vi "Mech Drive.vi"(11 "JoystickDevRef":T1) -> (3 "motor values":dbl[](array[numeric]))   [LabVIEW 2018]
uses:
  <vilib>/Rock Robotics/WPI/Joystick/WPI_JoystickDevRef.ctl
  <vilib>/Rock Robotics/WPI/Joystick/WPI_JoystickDeviceEnum.ctl
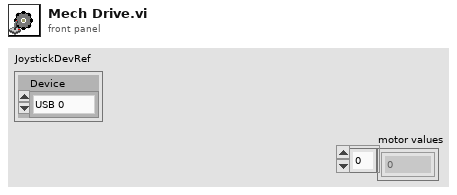
[diagram p1: front panel]
types:
  T1 = typedef "WPI_JoystickDevRef.ctl" = cluster{"Device":T2}
  T2 = typedef "WPI_JoystickDeviceEnum.ctl" = enum16{"USB 0", "USB 1", "USB 2", "USB 3", "USB 4", "USB 5"}
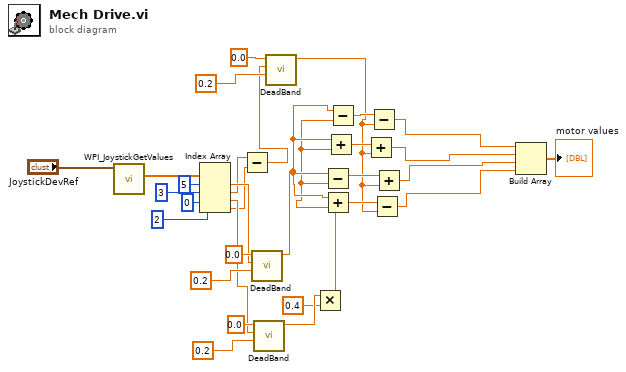
[diagram p0: block diagram]
diagram:
  n1 = call <vilib>:"WPI_JoystickGetValues.vi"("JoystickDevRef"="JoystickDevRef") -> ("Axes"=w30:dbl[])  [unwired: 6 in, 4 out]
  n2 = Index Array(array=w30, index #1=5 ("index"), index #2=3 ("index"), index #3=0 ("index"), index #4=2 ("index")) -> (element #1=w11:dbl, element #2=w7:dbl, element #3=w10:dbl, element #4=w6:dbl)
  n3 = Subtract(x=w7, y=w6) -> (x-y=w5:dbl)
  n4 = call "DeadBand.vi"("Threshold"=0.2, "Process Variable"=w11, "Send Value"=0.0) -> ("Output"=w4:dbl)  [unwired: 7 in, 1 out]
  n5 = call "DeadBand.vi"("Threshold"=0.2, "Process Variable"=w10, "Send Value"=0.0) -> ("Output"=w2:dbl)  [unwired: 7 in, 1 out]
  n6 = call "DeadBand.vi"("Threshold"=0.2, "Process Variable"=w5, "Send Value"=0.0) -> ("Output"=w17:dbl)  [unwired: 7 in, 1 out]
  n7 = Multiply(x=w2, y=0.4) -> (x*y=w3:dbl)
  n8 = Subtract(x=w4, y=w3) -> (x-y=w25:dbl)
  n9 = Add(x=w4, y=w3) -> (x+y=w24:dbl)
  n10 = Add(x=w4, y=w3) -> (x+y=w26:dbl)
  n11 = Subtract(x=w4, y=w3) -> (x-y=w27:dbl)
  n12 = Add(x=w26, y=w17) -> (x+y=w22:dbl)
  n13 = Subtract(x=w27, y=w17) -> (x-y=w23:dbl)
  n14 = Subtract(x=w24, y=w17) -> (x-y=w20:dbl)
  n15 = Add(x=w25, y=w17) -> (x+y=w21:dbl)
  n16 = Build Array(w23, w22, w21, w20) -> (→"motor values":dbl[])
